vi "Day 21-Part 2.vi"() -> ()   [LabVIEW 2021]
uses:
  Day 21-Turn Cluster.ctl
  Day 21-Player Turn.ctl
panel:
  out "Time to Solve":dbl
  out "Player 2 Win Count":u64
  out "Player 1 Win Count":u64
  in  "Player 2 Starting Position":u64=3
  in  "Player 1 Starting Position":u64=10
  out "Maximum Score":u64
  # "Example:\nPlayer 1 starting position: 4\nPlayer 2 starting position: 8"
  # "Input:\nPlayer 1 starting position: 10\nPlayer 2 starting position: 3"
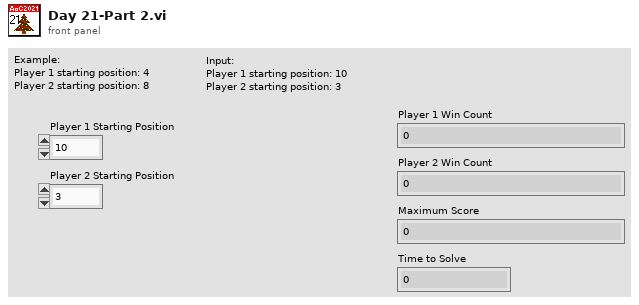
[diagram p1: front panel]
types:
  T1 = typedef "Day 21-Turn Cluster.ctl" = cluster{"Player 1 Position":u64, "Player 1 Score":u64, "Player 2 Position":u64, "Player 2 Score":u64, "Player Turn":T2}
  T2 = typedef "Day 21-Player Turn.ctl" = enum16{"Player 1", "Player 2"}
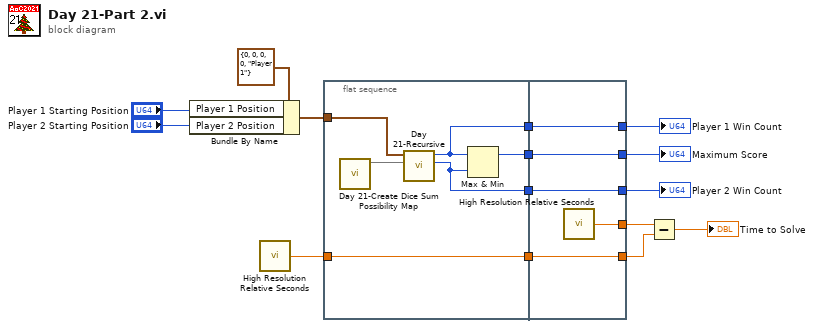
[diagram p0: block diagram]
diagram:
  n1 = Bundle By Name(cluster=T1 {"Player 1 Position"=0, "Player 1 Score"=0, "Player 2 Position"=0, "Player 2 Score"=0, "Player Turn"=enum."Player 1"}, "Player 1 Position"="Player 1 Starting Position", "Player 2 Position"="Player 2 Starting Position") -> (w11:T1)
  n2 = call <vilib>:"High Resolution Relative Seconds.vi"() -> ("relative seconds"=w5:dbl)
  n3 = flat-sequence {
    tunnel: w11 -> [w17]
    tunnel: [w21] -> w8
    tunnel: [w20] -> w7
    tunnel: [w19] -> w6
    tunnel: w5 -> [w16]
    tunnel: [w16] -> w4
    tunnel: [w24] -> w13
    tunnel: [w25] -> w14
    tunnel: [w26] -> w15
    tunnel: w8 -> [w26]
    tunnel: w7 -> [w25]
    tunnel: w6 -> [w24]
    tunnel: w4 -> [w22]
    tunnel: [w23] -> w3
    tunnel: [w22] -> w2
    frame #0 {
      n4 = call "Day 21-Create Dice Sum Possibility Map.vi"() -> ("Map"=w18:map{u64, u64})  [unwired: 11 in]
      n5 = call "Day 21-Recursive.vi"("Map"=w18, "State"=w17) -> ("Player 2 Win Count out"=w20:u64, "Player 1 Win Count out"=w21:u64)  [unwired: 8 in]
      n6 = Max & Min(x=w21, y=w20) -> (max(x,y)=w19:u64)  [unwired: 1 out]
    }
    frame #1 {
      n7 = call <vilib>:"High Resolution Relative Seconds.vi"() -> ("relative seconds"=w23:dbl)
    }
  }
  n8 = Subtract(x=w3, y=w2) -> (x-y=→"Time to Solve":dbl)
  "Maximum Score" <- w13
  "Player 1 Win Count" <- w15
  "Player 2 Win Count" <- w14
